vi "Set Cached Result.vi"(4 "Cached results":i32[](array[numeric]), 5 "Cacheable?":bool, 7 "Cache string":string, 8 "error in (no error)":errorcluster, 11 "Composite Object in":refnum<class "CConfig Object.lvclass">) -> (0 "error out":errorcluster, 3 "Composite Object out":refnum<class "CConfig Object.lvclass">)   [LabVIEW 2013, in "CConfig Object.lvclass"]
doc: "Copyright 2018, Carya Automatisering, Wiebe Walstra."
uses:
  CConfig Object.lvclass
  CConfig Object.lvclass/CConfig Object.ctl
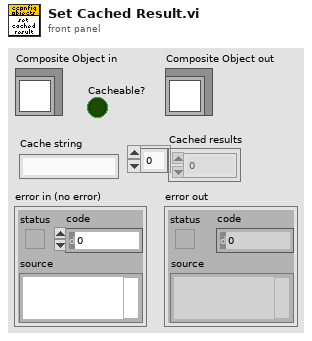
[diagram p1: front panel]
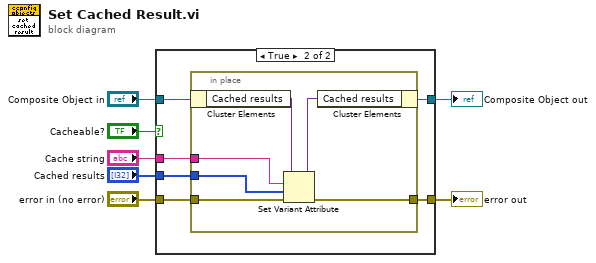
[diagram p0: block diagram]
diagram:
  n1 = case shown="True" "Cacheable?" {
    tunnel: "Composite Object in" -> [w9 w13]
    tunnel: [w9 w12] -> w6
    tunnel: "error in (no error)" -> [w8 w15]
    tunnel: [w8 w14] -> w4
    tunnel: "Cache string" -> [_ w11]
    tunnel: "Cached results" -> [_ w10]
    frame False {
    }
    frame True {
      n2 = in-place {
        in-place-border: w15 -> [w21]
        in-place-border: [w20] -> w14
        in-place-border: w11 -> [w17]
        in-place-border: w10 -> [w16]
        n3 = in-place-cluster #1(w13) -> ("Cached results"=w19:variant)
        n4 = Set Variant Attribute(Variant=w19, name=w17, value=w16, error in=w21) -> (Variant out=w18:variant, error out=w20:errorcluster)  [unwired: 1 out]
        n5 = in-place-cluster #1("Cached results"=w18) -> (w12:refnum<class "CConfig Object.lvclass">)
      }
    }
  }
  "error out" <- w4
  "Composite Object out" <- w6
